vi "StartPanel.vi"(8 "error in (no error)":errorcluster caption="Error In") -> (0 "error out":errorcluster caption="Error Out")   [LabVIEW 2020]
panel:
  out "Title":u8(slide) scale=0.0..100.0
  # "欢迎使用宁波拜特燃料电池测试系统"
  # "文件加载中请稍后..."
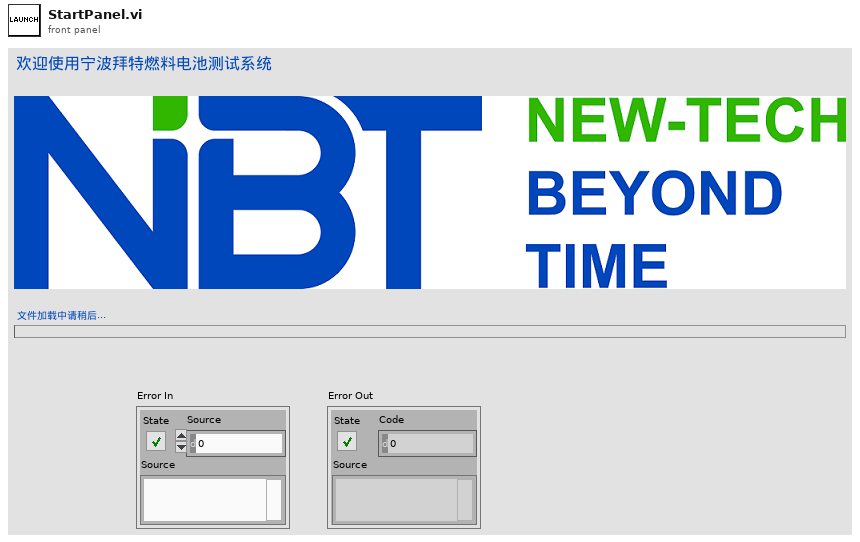
[diagram p1: front panel]
types:
  T1 = enum32{"Invalid", "Standard", "Closed", "Hidden", "Minimized", "Maximized"}
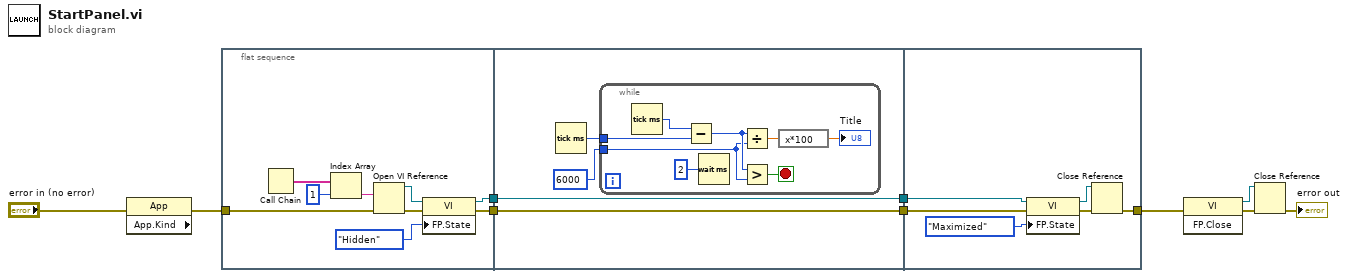
[diagram p0: block diagram]
diagram:
  n1 = property class="App" props=["App.Kind"](error in="error in (no error)") -> (error out=w7:errorcluster)  [unwired: 1 in, 2 out]
  n2 = flat-sequence {
    tunnel: [w14] -> w4
    tunnel: w7 -> [w12]
    tunnel: [w11] -> w3
    tunnel: w4 -> [w21]
    tunnel: [w21] -> w2
    tunnel: [w20] -> w1
    tunnel: w3 -> [w20]
    tunnel: w2 -> [w37]
    tunnel: [w33] -> w8
    tunnel: w1 -> [w32]
    frame #0 {
      n3 = Call Chain() -> (call chain=w18:string[])
      n4 = Index Array(array=w18, index=1 ("索引")) -> (element=w16:string)
      n5 = Open VI Reference(vi path=w16, error in (no error)=w12) -> (vi reference=w15:refnum<vi>, error out=w13:errorcluster)  [unwired: 4 in]
      n6 = property class="VI"(reference=w15, error in=w13, "FP.State"=T1."Hidden" ("前面板窗口:状态")) -> (reference out=w14:refnum<vi>, error out=w11:errorcluster)
    }
    frame #1 {
      n7 = Tick Count (ms)() -> (millisecond timer value=w23:u32)
      n8 = while {
        tunnel: w23 -> [w30]
        tunnel: 6000 -> [w26]
        stop <- w28 stop-if-true
        n9 = Tick Count (ms)() -> (millisecond timer value=w31:u32)
        n10 = Subtract(x=w31, y=w30) -> (x-y=w27:u32)
        n11 = Wait (ms)(milliseconds to wait=u32 2 ("等待时间（毫秒）")) -> ()  [unwired: 1 out]
        n12 = Divide(x=w27, y=w26) -> (x/y=w25:dbl)
        n13 = Greater?(x=w27, y=w26) -> (0:w28:bool)
        n14 = expression code="x*100"(w25) -> (→"Title":dbl)
      }
    }
    frame #2 {
      n15 = property class="VI"(reference=w37, error in=w32, "FP.State"=T1."Maximized" ("前面板窗口:状态")) -> (reference out=w34:refnum<vi>, error out=w35:errorcluster)
      n16 = Close Reference(reference=w34, error in (no error)=w35) -> (error out=w33:errorcluster)
    }
  }
  n17 = invoke class="VI" method="FP.Close"(error in=w8) -> (reference out=w10:refnum<vi>, error out=w9:errorcluster)  [unwired: 2 in, 1 out]
  n18 = Close Reference(reference=w10, error in (no error)=w9) -> (error out=→"error out":errorcluster)
